vi "gainLevels_errorCheck.vi"(8 "error in":errorcluster, 9 "search value":dbl, 10 "GainLevel array":dbl[](array[numeric]), 11 "gain levels nr max":u16) -> (0 "error out":errorcluster, 2 "gain levels active":dbl[](array[numeric]))   [LabVIEW 2010, in "OSA.lvclass"]
uses:
  OSA.lvclass
  OSA20X_misc.lvlib
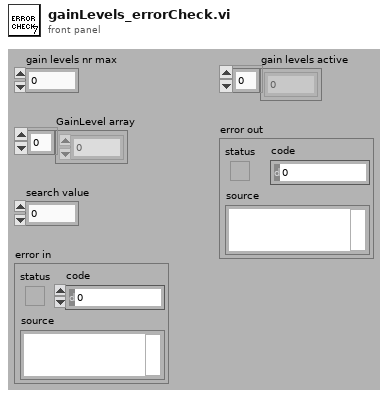
[diagram p1: front panel]
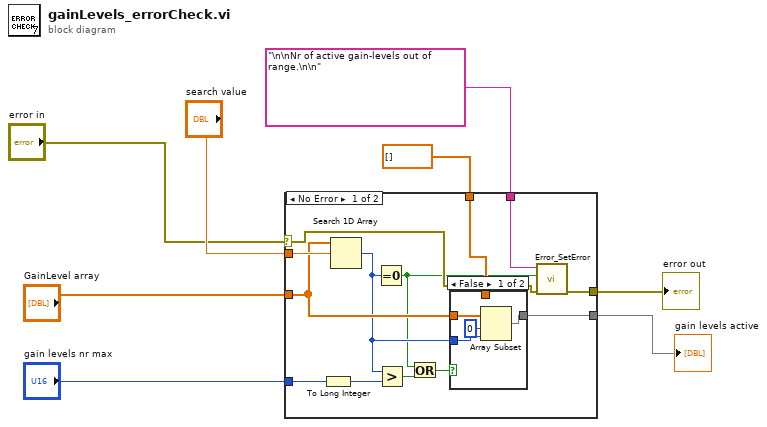
[diagram p0: block diagram]
diagram:
  n1 = case shown="No Error" "error in" {
    selector: "error in" -> [w12 w28]
    tunnel: "GainLevel array" -> [w18 _]
    tunnel: "search value" -> [w21 _]
    tunnel: "\n\nNr of active gain-levels out of range.\n\n" ("source(\"\")") -> [w20 _]
    tunnel: [w19 w28] -> w5
    tunnel: [w17 w27] -> w6
    tunnel: dbl[] [] -> [w16 w27]
    tunnel: "gain levels nr max" -> [w15 _]
    frame No Error {
      n2 = To Long Integer(number=w15) -> (32bit integer=w13:i32)
      n3 = Search 1D Array(1D array=w18, element=w21) -> (index of element=w14:i32)  [unwired: 1 in]
      n4 = Equal To 0?(x=w14) -> (x = 0?=w10:bool)
      n5 = Greater?(x=w14, y=w13) -> (0:w11:bool)
      n6 = Or(x=w10, y=w11) -> (x .or. y?=w9:bool)
      n7 = case shown="False" w9 {
        tunnel: w18 -> [w25 _]
        tunnel: w14 -> [w24 _]
        tunnel: [w22 w26] -> w17
        tunnel: w16 -> [_ w26]
        frame False {
          n8 = Array Subset(array=w25, index=0, length=w24) -> (w22:dbl[])
        }
        frame True {
        }
      }
      n9 = call "Error_SetError.vi"("error in"=w12, "status (true)"=w10, "source(\"\")"=w20) -> ("error out"=w19:errorcluster)  [unwired: 4 in]
    }
    frame Error {
    }
  }
  "gain levels active" <- w6
  "error out" <- w5
